vi "LNLS Control Encode BPM.vi"(8 "error in (no error)":errorcluster, 11 "BPM Data":T1[](array[typedef]) {"status" format="%08b"}) -> (0 "error out":errorcluster, 2 "command body":string)   [LabVIEW 2011, in "LNLS Control VIs.lvlib"]
uses:
  LNLS Control VIs.lvlib
  Types Definitions/Type BPM Pre Encode.ctl
  Type Definitions.lvlib
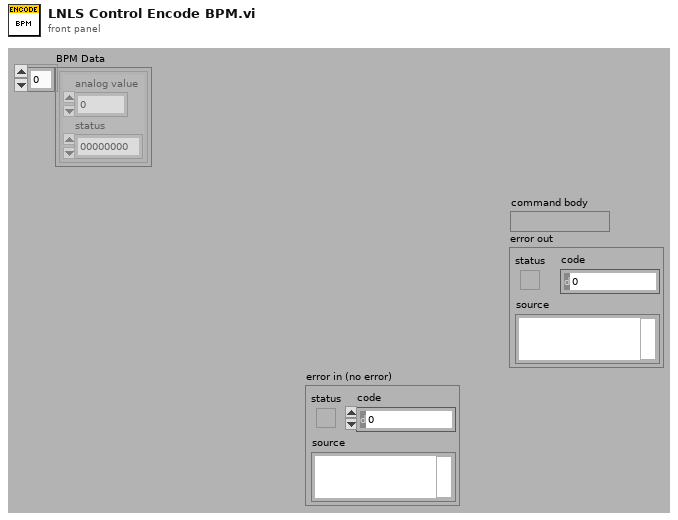
[diagram p1: front panel]
types:
  T1 = typedef "Type Definitions.lvlib/Type BPM Pre Encode.ctl" = cluster{"analog value":dbl, "status":u8}
  T2 = enum16{"big-endian, network order", "native, host order", "little-endian"}
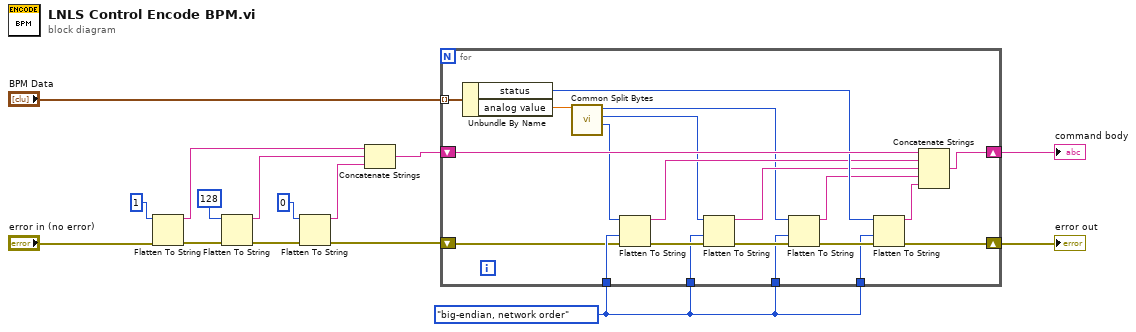
[diagram p0: block diagram]
diagram:
  w9 = T2."big-endian, network order" ("byte order (0:big-endian, network order)")
  n1 = Flatten To String(anything=u8 1 ("priority"), error in (no error)="error in (no error)") -> (data string=w7:string, error out=w13:errorcluster)  [unwired: 2 in, 1 out]
  n2 = Flatten To String(anything=u8 128 ("flag"), error in (no error)=w13) -> (data string=w6:string, error out=w3:errorcluster)  [unwired: 2 in, 1 out]
  n3 = Flatten To String(anything=u16 0 ("Number of Integrations"), error in (no error)=w3) -> (data string=w2:string, error out=w1:errorcluster)  [unwired: 2 in, 1 out]
  n4 = Concatenate Strings(w7, w6, w2) -> (w5:string)
  n5 = for {
    shift-right: [w32] -> w15
    shift-left: w1 -> [w25]
    tunnel: "BPM Data" -> [w34] mode=indexing
    shift-right: [w31] -> w14
    shift-left: w5 -> [w30]
    tunnel: w9 -> [w27]
    tunnel: w9 -> [w26]
    tunnel: w9 -> [w21]
    tunnel: w9 -> [w20]
    n6 = Unbundle By Name(w34) -> ("status"=w29:u8, "analog value"=w19:dbl)
    n7 = call "Common Split Bytes.vi"("Double"=w19) -> ("Most Significant Byte"=w18:u8, "Intermediate Byte"=w17:u8, "Less Significant Byte"=w16:u8)  [unwired: 8 in]
    n8 = Flatten To String(anything=w18, byte order (0:big-endian, network order)=w26, error in (no error)=w25) -> (data string=w28:string, error out=w33:errorcluster)  [unwired: 1 in, 1 out]
    n9 = Flatten To String(anything=w17, byte order (0:big-endian, network order)=w21) -> (data string=w23:string)  [unwired: 2 in, 2 out]
    n10 = Flatten To String(anything=w16, byte order (0:big-endian, network order)=w20) -> (data string=w22:string)  [unwired: 2 in, 2 out]
    n11 = Flatten To String(anything=w29, byte order (0:big-endian, network order)=w27, error in (no error)=w33) -> (data string=w24:string, error out=w32:errorcluster)  [unwired: 1 in, 1 out]
    n12 = Concatenate Strings(w30, w28, w23, w22, w24) -> (w31:string)
  }
  "command body" <- w14
  "error out" <- w15
